vi "Get Beacon Position.vi"(8 "Decision Point":u8=80, 10 "NXT":T1) -> (0 "IR Data":u8, 1 "f":i32, 2 "NXT Out":T1={"Hardware"="NXT", "Flattened String"=""})   [LabVIEW 2010, in "4150_RingItUp_State.lvrbt"]
uses:
  4150_RingItUp_State/4150_RingItUp_State.lvrbt
  <vilib>/NXT/Subs/LVHSConnector.ctl
  <vilib>/NXT/HiTechnic/HiTechnic Controls/HiTechnic Port.ctl
  <vilib>/NXT/Block Support/NXT_InputPort.ctl
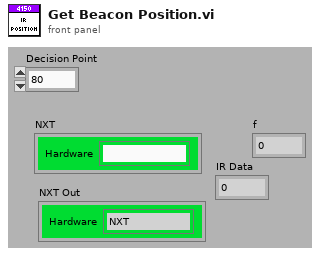
[diagram p1: front panel]
types:
  T1 = typedef "LVHSConnector.ctl" = cluster{"Hardware":string, "Flattened String":string}
  T2 = typedef "HiTechnic Port.ctl" = cluster{"Port":T3, "MUX Port":u8}
  T3 = typedef "NXT_InputPort.ctl" = u8
  T4 = cluster{"Direction (0-9)":i16, "Signal Strength (Array)":u8[]}
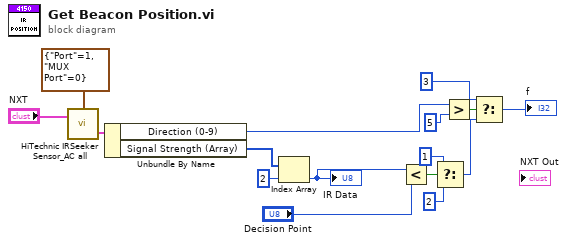
[diagram p0: block diagram]
diagram:
  n1 = call <vilib>:"HiTechnic IRSeeker Sensor_AC all.vi"("NXT"="NXT", "Port/MUX"=T2 {"Port"=1, "MUX Port"=0}) -> ("All Info"=w2:T4)  [unwired: 1 in, 1 out]
  n2 = Unbundle By Name(w2) -> ("Direction (0-9)"=w5:i16, "Signal Strength (Array)"=w3:u8[])
  n3 = Index Array(array=w3, index=2) -> (element=w10:u8)
  "IR Data" <- w10
  n4 = Less?(x=w10, y="Decision Point") -> (x < y?=w9:bool)
  n5 = Select(t=1, s=w9, f=2) -> (s? t:f=w14:i32)
  n6 = Greater?(x=w5, y=i16 5) -> (0:w6:bool)
  n7 = Select(t=3, s=w6, f=w14) -> (s? t:f=→"f":i32)
